vi "SquareWaveGenerato.vi"(4 "Sampling Period":dbl, 6 "phase":dbl, 7 "Iteration Count":i32, 8 "Noise Std":dbl=1.0 format="%0.2f", 9 "amplitude":dbl, 10 "frequency":dbl, 11 "Number of Samples":i32) -> (3 "Array":dbl[](array[numeric]))   [LabVIEW 2019]
uses:
  <vilib>/ptbypt/NI_PtbyPt.lvlib
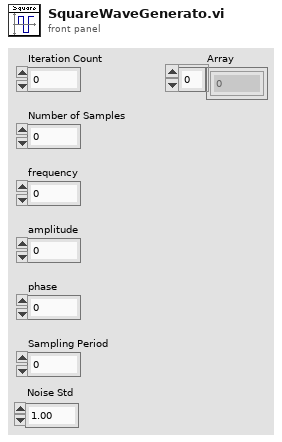
[diagram p1: front panel]
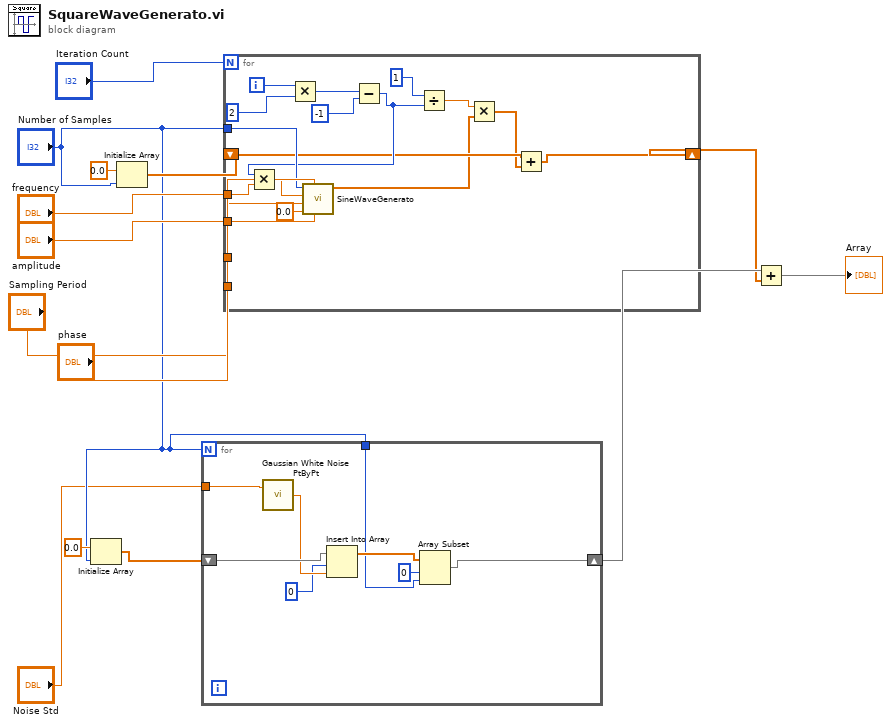
[diagram p0: block diagram]
diagram:
  n1 = Initialize Array(0.0 ("element"), "Number of Samples") -> (w7:dbl[])
  n2 = Initialize Array(0.0 ("element"), "Number of Samples") -> (w11:dbl[])
  n3 = for {
    N: "Number of Samples" -> [_]
    shift-right: [w15] -> w5
    shift-left: w7 -> [w21]
    tunnel: "Noise Std" -> [w22]
    tunnel: "Number of Samples" -> [w16]
    n4 = call <vilib>:"Gaussian White Noise PtByPt.vi"("standard deviation"=w22) -> ("Gaussian white noise"=w20:dbl)  [unwired: 2 in]
    n5 = Insert Into Array(array=w21, index=0, new element=w20) -> (w18:dbl[])
    n6 = Array Subset(array=w18, index=0, length=w16) -> (w15:dbl[])
  }
  n7 = for {
    N: "Iteration Count" -> [_]
    shift-right: [w23] -> w4
    shift-left: w11 -> [w29]
    tunnel: "Sampling Period" -> [w34]
    tunnel: "frequency" -> [w31]
    tunnel: "Number of Samples" -> [w33]
    tunnel: "phase" -> [w27]
    tunnel: "amplitude" -> [w26]
    i -> [w40]
    n8 = Multiply(x=w40, y=2) -> (x*y=w38:i32)
    n9 = Subtract(x=w38, y=-1 ("x*y")) -> (x-y=w32:i32)
    n10 = Multiply(x=w32, y=w31) -> (x*y=w30:dbl)
    n11 = call "SineWaveGenerato.vi"("amplitude"=w26, "Sampling Period"=w34, "Noise Std"=0.0, "phase"=w27, "frequency"=w30, "Number of Samples"=w33) -> ("Array"=w25:dbl[])  [unwired: 5 in]
    n12 = Divide(x=1, y=w32) -> (x/y=w35:dbl)
    n13 = Multiply(x=w35, y=w25) -> (x*y=w28:dbl[])
    n14 = Add(x=w29, y=w28) -> (x+y=w23:dbl[])
  }
  n15 = Add(x=w5, y=w4) -> (x+y=→"Array":dbl[])
